vi "save scale.vi"(7 "Index":u32) -> (0 "error":errorcluster)   [LabVIEW 2012]
uses:
  DAC project/Calibration and Function folders.ctl
  calibration/global scale array.vi
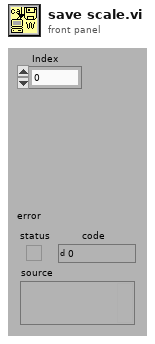
[diagram p1: front panel]
types:
  T1 = typedef "Calibration and Function folders.ctl" = enum16{"Sensors", "Functions", "Config File", "UserAppFolder"}
  T2 = enum16{"open", "open or create", "create or replace", "create", "open (read only)"}
  T3 = typedef "calib array.ctl" = T4[]
  T4 = typedef "conversion.ctl" = cluster{"conversion matrix":sgl[][], "units":string, "name":string, "scale type":T5, "offset (volts)":dbl, "second channel":i8, "correspondence table":T6, "offset (physical units)":dbl, "pH scale":T7, "D.O.":T8}
  T5 = typedef "scale type.ctl" = enum16{"Volts", "Polynomial", "Correspondence Table", "pH", "Dissolved Oxygen", "Quadratic"}
  T6 = typedef "correspondence table.ctl" = cluster{"physical units":dbl, "volts":dbl}[]
  T7 = typedef "pH scale.ctl" = cluster{"Buffers":cluster{"Buffer":dbl, "Calibrated":bool, "V/T":dbl}[], "Temperature":dbl}
  T8 = typedef "DO scale.ctl" = cluster{"Temperature":dbl, "K":dbl, "barometric pressure":dbl}
  T9 = enum16{"open", "replace", "create", "open or create", "replace or create", "replace or create with confirmation"}
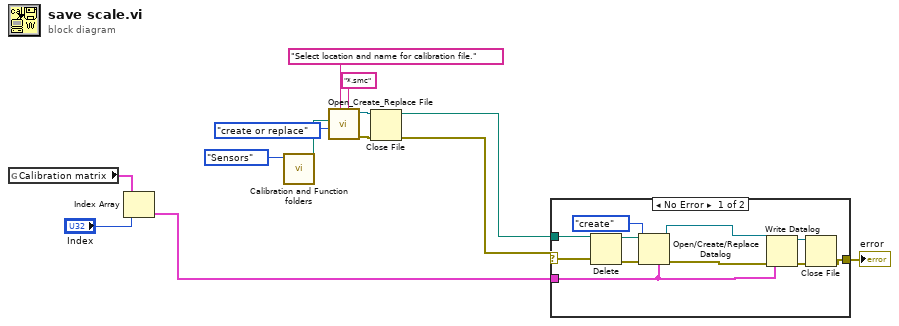
[diagram p0: block diagram]
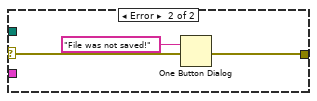
[diagram p2: hidden frame]
diagram:
  n1 = global read "global scale array.vi" "Calibration matrix"() -> (w6:T3)
  n2 = Index Array(array=w6, index="Index") -> (element=w3:T4)
  n3 = call "Calibration and Function folders.vi"("Folder"=Calibration_and_Function_folders."Sensors") -> ("Selected Folder"=w2:path)  [unwired: 10 in]
  n4 = call <vilib>:"Open_Create_Replace File.vi"("pattern"="*.smc", "prompt"="Select location and name for calibration file.", "function (open:0)"=T2."create or replace", "start path  (Not A Path)"=w2) -> ("error out"=w11:errorcluster, "refnum"=w10:refnum<file>)  [unwired: 4 in, 2 out]
  n5 = Close File(refnum=w10, error in=w11) -> (path=w4:path, error out=w7:errorcluster)
  n6 = case shown="No Error" w7 {
    selector: w7 -> [w18 w25]
    tunnel: w4 -> [w16 _]
    tunnel: w3 -> [w21 _]
    tunnel: [w22 w25] -> w8
    frame No Error {
      n7 = Delete(path (use dialog)=w16, error in=w18) -> (deleted path=w15:path, error out=w17:errorcluster)  [unwired: 3 in, 1 out]
      n8 = Open/Create/Replace Datalog(5:w21, 8:w17, 10:T9."create" ("operation (0:open)"), 11:w15) -> (0:w19:errorcluster, 3:w20:refnum<k1>)  [unwired: 2 in, 1 out]
      n9 = Write Datalog(4:w19, 6:w21, 7:w20) -> (0:w24:errorcluster, 3:w23:refnum<k1>)
      n10 = Close File(refnum=w23, error in=w24) -> (error out=w22:errorcluster)  [unwired: 1 out]
    }
    frame Error {
      n11 = One Button Dialog(message="File was not saved!") -> ()  [unwired: 1 in, 1 out]
    }
  }
  "error" <- w8
